vi "子VI-修改评定结果.vi"(9 "全部检测结果":string[][](table), 11 "临界面积百分比值":dbl) -> (1 "全部检测结果合并输出":string[][](table) caption="全部检测结果")   [LabVIEW 2018]
panel:
  in  "ok":bool
  in  "确定按钮":bool
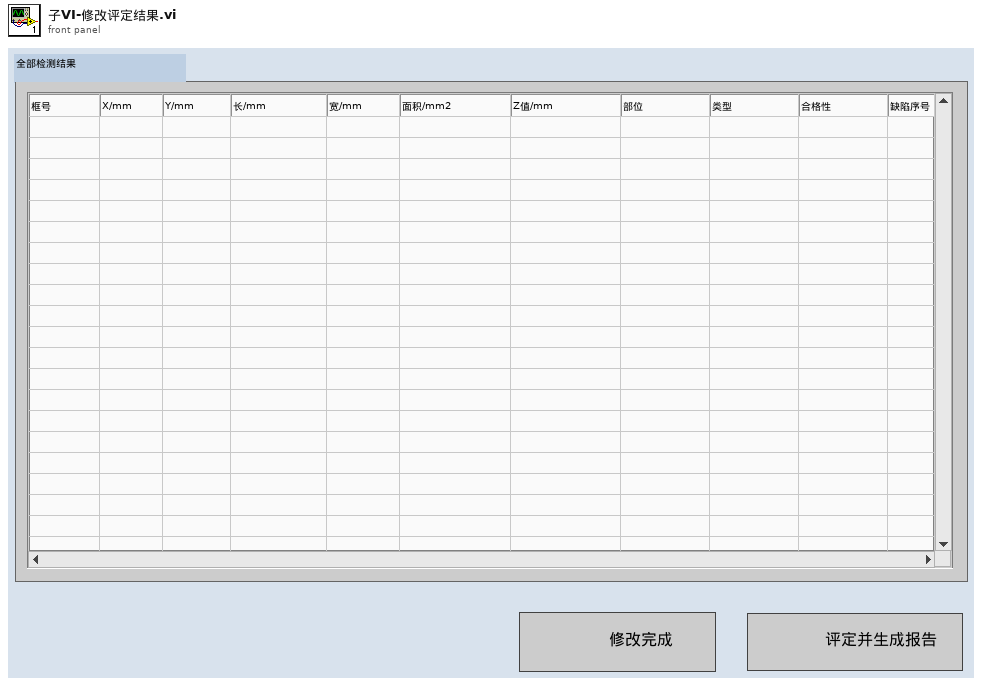
[diagram p1: front panel]
types:
  T1 = enum8{"Enabled", "Disabled", "Disabled and Grayed Out"}
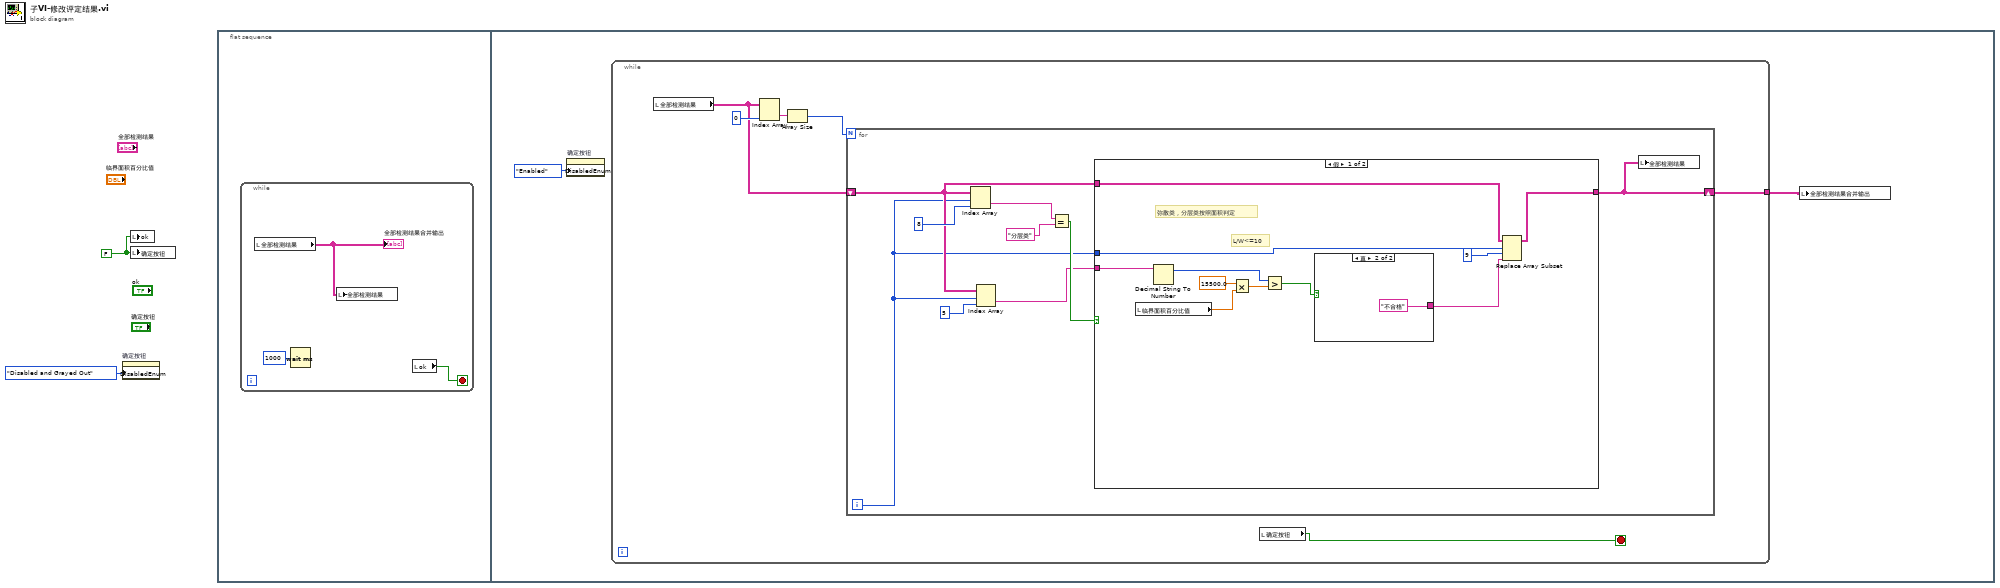
[diagram p0: block diagram]
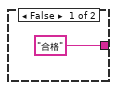
[diagram p2: hidden frame]
diagram:
  w2 = FALSE
  n1 = property on="确定按钮" class="Bool (严格)"("DisabledEnum"=T1."Disabled and Grayed Out" ("禁用")) -> ()  [unwired: 2 in, 2 out]
  n2 = local write "ok"(w2) -> ()
  n3 = local write "确定按钮"(w2) -> ()
  n4 = flat-sequence {
    frame #0 {
      n5 = while {
        stop <- w3 stop-if-true
        n6 = local read "全部检测结果"() -> (w4:string[][])
        "全部检测结果合并输出" <- w4
        n7 = Wait (ms)(milliseconds to wait=u32 1000 ("等待时间（毫秒）")) -> ()  [unwired: 1 out]
        n8 = local write "全部检测结果"(w4) -> ()
        n9 = local read "ok"() -> (w3:bool)
      }
    }
    frame #1 {
      n10 = property on="确定按钮" class="Bool (严格)"("DisabledEnum"=T1."Enabled" ("禁用")) -> ()  [unwired: 2 in, 2 out]
      n11 = while {
        tunnel: [w8] -> w6
        stop <- w12 stop-if-true
        n12 = local read "全部检测结果"() -> (w9:string[][])
        n13 = Index Array(array=w9, index (col)=0 ("禁用的索引 (列)")) -> (element=w10:string[])  [unwired: 1 in]
        n14 = Array Size(array=w10) -> (size(s)=w13:i32)
        n15 = for {
          N: w13 -> [_]
          shift-right: [w14] -> w8
          shift-left: w9 -> [w18]
          i -> [w17]
          n16 = Index Array(array=w18, index (row)=w17, index (col)=8 ("禁用的索引 (列)")) -> (element=w20:string)
          n17 = Index Array(array=w18, index (row)=w17, index (col)=5 ("禁用的索引 (列)")) -> (element=w15:string)
          n18 = Equal?(x=w20, y="分层类") -> (x = y?=w19:bool)
          n19 = case shown="假" w19 {
            tunnel: w18 -> [w30 w36]
            tunnel: w17 -> [w29 _]
            tunnel: [w26 w36] -> w14
            tunnel: w15 -> [w24 _]
            frame False {
              # "L/W<=10"
              # "弥散类，分层类按照面积判定"
              n20 = local read "临界面积百分比值"() -> (w31:dbl)
              n21 = Decimal String To Number(string=w24) -> (offset past number=w23:i32)  [unwired: 2 in, 1 out]
              n22 = Multiply(x=15500.0, y=w31) -> (x*y=w33:dbl)
              n23 = Greater?(x=w23, y=w33) -> (0:w25:bool)
              n24 = case shown="真" w25 {
                tunnel: ["合格" "不合格"] -> w27
                frame False {
                }
                frame True {
                }
              }
              n25 = Replace Array Subset(array=w30, new element=w27, index (row)=w29, index (col)=9 ("禁用的索引 (列)")) -> (w26:string[][])
            }
            frame True {
              # "分层类，合格性按照Z值\n默认不变"
            }
          }
          n26 = local write "全部检测结果"(w14) -> ()
        }
        n27 = local read "确定按钮"() -> (w12:bool)
      }
      n28 = local write "全部检测结果合并输出"(w6) -> ()
    }
  }
